vi "RSZVB Get Power Coeficients.vi"(8 "error in (no error)":errorcluster {"code" format="%.0x"}, 10 "Port (1)":i32=1, 11 "VISA session":refnum<visa-resource-name>) -> (0 "error out":errorcluster {"code" format="%.0x"}, 1 "Coeficients":dbl[](array[numeric]) format="%^.3e", 3 "dup VISA session":refnum<visa-resource-name>)   [LabVIEW 2011]
doc: "Returns power coefficients for frequency converters R&S ZVA-ZxxxE\n\nNotes:\n\n(1) This command is available for frequency converters with electronic attenuators R&S ZVA-ZxxxE.\n\nRemote-control command(s):\n[SENSe<Ch>:]FREQuency:CONVersion:DEVice:PCOefficient<Port>?"
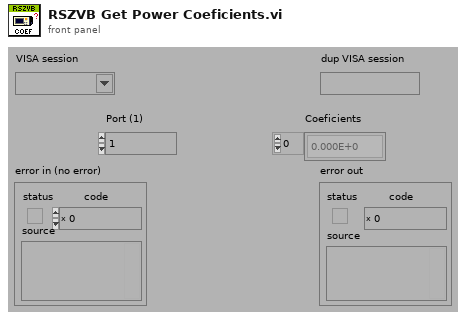
[diagram p1: front panel]
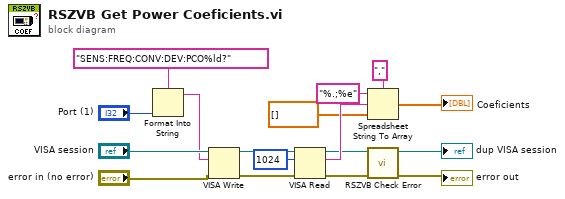
[diagram p0: block diagram]
diagram:
  n1 = Format Into String(format string="SENS:FREQ:CONV:DEV:PCO%ld?", "Port (1)") -> (resulting string=w13:string)  [unwired: 2 in, 1 out]
  n2 = VISA Write(VISA resource name="VISA session", write buffer=w13, error in (no error)="error in (no error)") -> (VISA resource name out=w11:refnum<visa-resource-name>, error out=w12:errorcluster)  [unwired: 1 out]
  n3 = VISA Read(VISA resource name=w11, byte count=u32 1024, error in (no error)=w12) -> (VISA resource name out=w5:refnum<visa-resource-name>, read buffer=w9:string, error out=w6:errorcluster)  [unwired: 1 out]
  n4 = Spreadsheet String To Array(delimiter (Tab)=",", format string="%.;%e", spreadsheet string=w9, array type (2D Dbl)=dbl[] []) -> (array=→"Coeficients":dbl[])
  n5 = call "RSZVB Check Error.vi"("error in (no error)"=w6, "VISA session"=w5) -> ("error out"=→"error out":errorcluster, "dup VISA session"=→"dup VISA session":refnum<visa-resource-name>)  [unwired: 8 in]
